vi "HVBuncher.UnloadObjects.vi"(0 "i ref in":refnum<vi>, 1 "ObjectsLoaded in":string[](array[string]), 5 "error in (no error)":errorcluster) -> (14 "i ref out":refnum<vi>, 15 "ObjectsLoaded out":string[](array[string]), 19 "error out":errorcluster)   [LabVIEW 2014, in "HVBuncher.lvlib"]
doc: "Unloads all objects specified."
uses:
  HVBuncher.lvlib
  CS_Core/CSSystem/CoreLib/CoreLib.string 2 byte array.vi
  CS_Core/CSSystem/CoreLib/CoreLib.lvlib
  CS_Core/BaseProcess/BaseProcess.lvlib
  CS_Core/CSSystem/CSSystemLib/CSSystemLib.lvlib
panel:
  in  "emptyArray":string[](array[string])
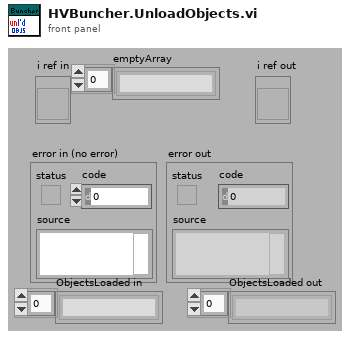
[diagram p1: front panel]
types:
  T1 = typedef "CoreDefs.rawDataType.ctl" = i8[]
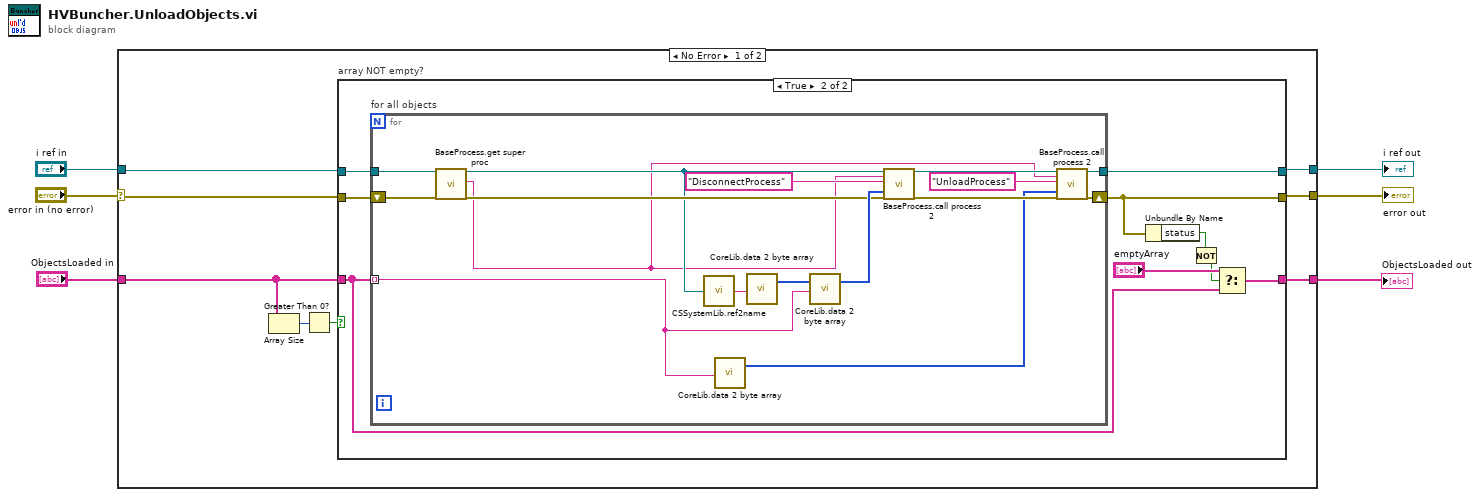
[diagram p0: block diagram]
diagram:
  n1 = case shown="No Error" "error in (no error)" {
    selector: "error in (no error)" -> [w7 w44]
    tunnel: [w14 w45] -> w6
    tunnel: [w13 w44] -> w5
    tunnel: "i ref in" -> [w8 w45]
    tunnel: "ObjectsLoaded in" -> [w9 w43]
    tunnel: [w10 w43] -> w1
    frame No Error {
      n2 = Array Size(array=w9) -> (size(s)=w12:i32)
      n3 = Greater Than 0?(x=w12) -> (x > 0?=w11:bool)
      n4 = case "array NOT empty?" shown="True" w11 {
        tunnel: w9 -> [w15 w22]
        tunnel: w8 -> [w17 w26]
        tunnel: w7 -> [w16 w25]
        tunnel: [w17 w24] -> w14
        tunnel: [w16 w23] -> w13
        tunnel: [w15 w20] -> w10
        frame False {
        }
        frame True {
          n5 = for "for all objects" {
            tunnel: w22 -> [w27] mode=indexing
            tunnel: [w42] -> w24
            shift-right: [w41] -> w23
            shift-left: w25 -> [w31]
            tunnel: w26 -> [w32]
            n6 = call "BaseProcess.get super proc.vi"("i ref in"=w32, "error in (no error)"=w31) -> ("i ref out"=w29:refnum<vi>, "SuperProc"=w28:string, "error out"=w30:errorcluster)  [unwired: 15 in]
            n7 = call "CSSystemLib.ref2name.vi"("obj refnum"=w29) -> ("name"=w35:string)
            n8 = call-poly "CoreLib.data 2 byte array.vi"("string"=w27) -> ("byteArray out"=w36:T1)  [unwired: 18 in]
            n9 = call-poly "CoreLib.data 2 byte array.vi"("string"=w35) -> ("byteArray out"=w34:T1)  [unwired: 18 in]
            n10 = call-poly "CoreLib.data 2 byte array.vi"("byteArray"=w34, "string"=w27) -> ("byteArray out"=w33:T1)  [unwired: 17 in]
            n11 = call "BaseProcess.call process 2.vi"("i ref in"=w29, "Object"=w28, "Selector"="DisconnectProcess", "Data"=w33, "error in (no error)"=w30) -> ("i ref out"=w40:refnum<vi>, "error out"=w39:errorcluster)  [unwired: 13 in]
            n12 = call "BaseProcess.call process 2.vi"("i ref in"=w40, "Object"=w28, "Selector"="UnloadProcess", "Data"=w36, "error in (no error)"=w39) -> ("i ref out"=w42:refnum<vi>, "error out"=w41:errorcluster)  [unwired: 13 in]
          }
          n13 = Unbundle By Name(w23) -> ("status"=w19:bool)
          n14 = Not(x=w19) -> (.not. x?=w18:bool)
          n15 = Select(t="emptyArray", s=w18, f=w22) -> (s? t:f=w20:string[])
        }
      }
    }
    frame Error {
    }
  }
  "error out" <- w5
  "i ref out" <- w6
  "ObjectsLoaded out" <- w1
